vi "test_Create MetaData Channel_array enumerated list.vi"(8 "error in (no error)":errorcluster, 11 "TestCase in":refnum<class "Instrument Addon Scripting API Channels Unit Tests.lvclass">) -> (0 "error out":errorcluster, 3 "TestCase out":refnum<class "Instrument Addon Scripting API Channels Unit Tests.lvclass">)   [LabVIEW 2019, in "Instrument Addon Scripting API Channels Unit Tests.lvclass"]
uses:
  Instrument Addon Scripting API Channels Unit Tests.lvclass
  Addon/Addon Shared/Types/FG Control.ctl
  APIs/Scripting API/TypeDefs/Array Enumerated List Settings.ctl
  APIs/Scripting API/TypeDefs/Array Element.ctl
  Instrument Addon Scripting API Channels Unit Tests.lvclass/Instrument Addon Scripting API Channels Unit Tests.ctl
  Addon/Addon Shared/SubVIs/Constants.vi
  <vilib>/NI VeriStand/Custom Device Tools/Custom Device Utility Library/NI VeriStand - Search for Item by Name.vi
  <vilib>/NI VeriStand/Custom Device API/NI VeriStand - Get Item Property.vi
  <vilib>/NI VeriStand/Custom Device API/Get Item Property (U32).vi
  <vilib>/NI VeriStand/Custom Device API/Get Item Property (String Array).vi
  <vilib>/NI VeriStand/Custom Device API/Get Item Property (String).vi
  <vilib>/NI VeriStand/Custom Device API/NI VeriStand - Set Item Property.vi
  <vilib>/NI VeriStand/Custom Device API/Set Item Property (U32).vi
  <vilib>/NI VeriStand/Custom Device API/Set Item Property (String Array).vi
  <vilib>/NI VeriStand/Custom Device API/NI VeriStand - Get Item Children.vi
  Addon/Addon Shared/SubVIs/Set Channel Value Table.vi
  <vilib>/NI VeriStand/Custom Device API/Set Item Property (String).vi
  <vilib>/NI VeriStand/Custom Device Tools/Custom Device Utility Library/NI VeriStand - Search for Item by GUID.vi
  APIs/Scripting API/Channels/Create MetaData Channel - Array - Enumerated List.vi
  <vilib>/addons/_JKI Toolkits/VI Tester/TestCase.llb/TestCase.lvclass
  <vilib>/NI VeriStand/Custom Device Tools/Custom Device Utility Library/Custom Device Utility Library.lvlib
  Addon/Addon Shared/Instrument Addon Shared.lvlib
  APIs/Scripting API/Instrument Addon Scripting API.lvlib
  C:/Program Files (x86)/National Instruments/LabVIEW 2019/vi.lib/addons/_JKI Toolkits/VI Tester/TestCase.llb/TestCase.lvclass
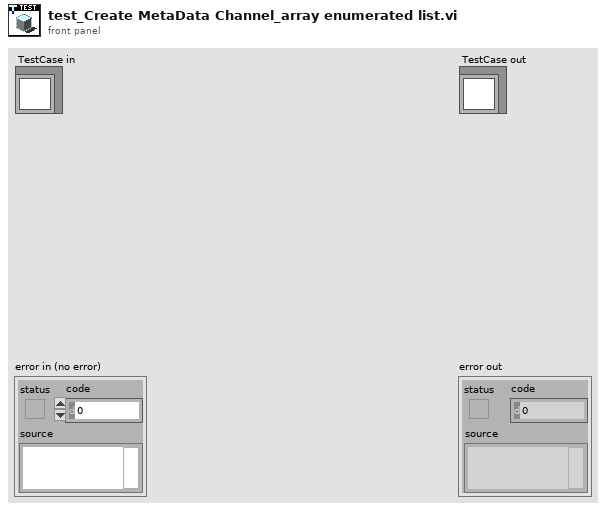
[diagram p1: front panel]
types:
  T1 = typedef "Instrument Addon Shared.lvlib/FG Control.ctl" = enum16{"Get", "Set"}
  T2 = typedef "Instrument Addon Scripting API.lvlib/Array Enumerated List Settings.ctl" = cluster{"Elements":T3[], "Enumerated List":string[], "Delimiter":string}
  T3 = typedef "Instrument Addon Scripting API.lvlib/Array Element.ctl" = cluster{"Name":string, "Default Value":dbl, "Units":string}
  T4 = typedef "Custom Device API.lvlib/Custom Device Item Ref.ctl" = u64
  T5 = typedef "Instrument Addon Shared.lvlib/MetaData Parameters.ctl" = cluster{"Data Type":T6, "Channel Type":T7, "List":string[], "Format String":string, "Type":T8, "Delimiter":string, "Endian":T9}
  T6 = typedef "Instrument Addon Shared.lvlib/Protocol Data Type.ctl" = enum16{"Single Channel", "Array"}
  T7 = typedef "Instrument Addon Shared.lvlib/Metadata Channel Type.ctl" = enum16{"Enumerated List", "Format", "Type Cast"}
  T8 = typedef "Instrument Addon Shared.lvlib/Type Cast Type.ctl" = enum16{"DBL", "SGL", "U64", "U32", "U16", "U8", "I64", "I32", "I16", "I8"}
  T9 = typedef "Instrument Addon Shared.lvlib/Endian.ctl" = enum16{"Native", "Little", "Big"}
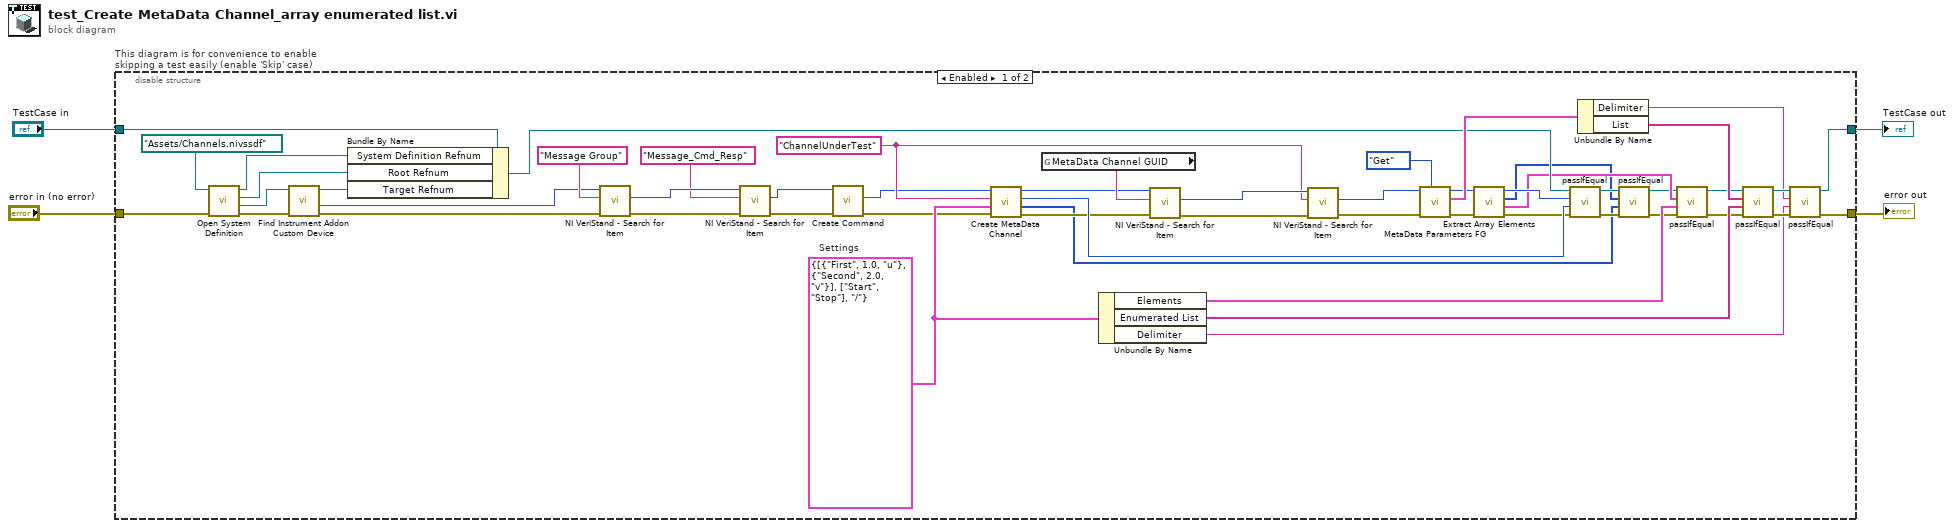
[diagram p0: block diagram]
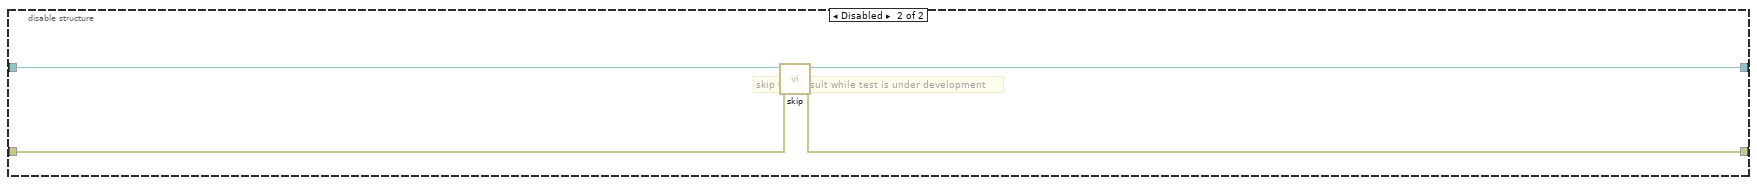
[diagram p2: hidden frame]
diagram:
  n1 = disable-structure "This diagram is for convenience to enable skipping a test easily (enable 'Skip' case)" shown="Enabled" {
    disable-tunnel: "TestCase in" -> [w39 w61]
    disable-tunnel: [w31 w59] -> w1
    disable-tunnel: [w30 w60] -> w3
    disable-tunnel: "error in (no error)" -> [w57 w58]
    frame Enabled {
      w34 = T2 {"Elements"=[{"Name"="First", "Default Value"=1.0, "Units"="u"}, {"Name"="Second", "Default Value"=2.0, "Units"="v"}], "Enumerated List"=["Start", "Stop"], "Delimiter"="/"}  # Settings
      w38 = "ChannelUnderTest" ("Name")
      n2 = call "Open System Definition.vi"("error in (no error)"=w57, "System Definition File"=path "Assets/Channels.nivssdf") -> ("error out"=w55:errorcluster, "Target Refnum"=w56:refnum<k24>, "Root Refnum"=w42:refnum<k24>, "System Definition Refnum"=w41:refnum<k24>)  [unwired: 6 in]
      n3 = call "Find Instrument Addon Custom Device.vi"("error in"=w55, "target in"=w56) -> ("error out"=w17:errorcluster, "NodeID"=w18:u64, "target out"=w43:refnum<k24>)  [unwired: 7 in]
      n4 = Bundle By Name(cluster=w39, "System Definition Refnum"=w41, "Root Refnum"=w42, "Target Refnum"=w43) -> (w40:refnum<class "Instrument Addon Scripting API Channels Unit Tests.lvclass">)
      n5 = call-poly <vilib>:"NI VeriStand - Search for Item.vi"("error in"=w17, "Item Name"="Message Group", "Section Ref in"=w18) -> ("error out"=w19:errorcluster, "Item Ref"=w21:T4)  [unwired: 5 in, 2 out]
      n6 = call-poly <vilib>:"NI VeriStand - Search for Item.vi"("error in"=w19, "Item Name"="Message_Cmd_Resp", "Section Ref in"=w21) -> ("error out"=w8:errorcluster, "Item Ref"=w7:T4)  [unwired: 5 in, 2 out]
      n7 = call "Create Command.vi"("error in"=w8, "message refnum In"=w7) -> ("error out"=w5:errorcluster, "command refnum"=w6:T4)  [unwired: 7 in, 1 out]
      n8 = call-poly "Create MetaData Channel.vi"("error in (no error)"=w5, "settings"=w34, "channel name"=w38, "command refnum in"=w6) -> ("error out"=w35:errorcluster, "channel refnums"=w10:T4[], "array refnum"=w36:T4, "command refnum out"=w37:T4)  [unwired: 4 in]
      n9 = global read "Constants.vi" "MetaData Channel GUID"() -> (w54:string)
      n10 = Unbundle By Name(w34) -> ("Elements"=w27:T3[], "Enumerated List"=w44:string[], "Delimiter"=w33:string)
      n11 = call-poly <vilib>:"NI VeriStand - Search for Item.vi"("error in"=w35, "Item GUID"=w54, "Section Ref in"=w37) -> ("error out"=w52:errorcluster, "Item Ref"=w53:T4)  [unwired: 5 in, 2 out]
      n12 = call-poly <vilib>:"NI VeriStand - Search for Item.vi"("error in"=w52, "Item Name"=w38, "Section Ref in"=w53) -> ("error out"=w51:errorcluster, "Item Ref"=w50:T4)  [unwired: 5 in, 2 out]
      n13 = call "MetaData Parameters FG.vi"("Action"=FG_Control."Get", "error in (no error)"=w51, "Item Ref in"=w50) -> ("error out"=w26:errorcluster, "MetaData Parameters"=w48:T5, "Item Ref out"=w25:T4)  [unwired: 6 in]
      n14 = call "Extract Array Elements.vi"("error in (no error)"=w26, "array reference in"=w25) -> ("error out"=w24:errorcluster, "elements"=w16:T3[], "channel refnums"=w11:T4[], "array reference out"=w23:T4)  [unwired: 6 in]
      n15 = call-dynamic "passIfEqual.vi"("error in (no error)"=w24, "y"=w36, "x"=w23, "TestCase in"=w40) -> ("error out"=w14:errorcluster, "TestCase out"=w15:refnum<class "Instrument Addon Scripting API Channels Unit Tests.lvclass">)  [unwired: 6 in]
      n16 = Unbundle By Name(w48) -> ("Delimiter"=w32:string, "List"=w45:string[])
      n17 = call-dynamic "passIfEqual.vi"("error in (no error)"=w14, "y"=w10, "x"=w11, "TestCase in"=w15) -> ("error out"=w13:errorcluster, "TestCase out"=w12:refnum<class "Instrument Addon Scripting API Channels Unit Tests.lvclass">)  [unwired: 6 in]
      n18 = call-dynamic "passIfEqual.vi"("error in (no error)"=w13, "y"=w27, "x"=w16, "TestCase in"=w12) -> ("error out"=w28:errorcluster, "TestCase out"=w29:refnum<class "Instrument Addon Scripting API Channels Unit Tests.lvclass">)  [unwired: 6 in]
      n19 = call-dynamic "passIfEqual.vi"("error in (no error)"=w28, "y"=w44, "x"=w45, "TestCase in"=w29) -> ("error out"=w47:errorcluster, "TestCase out"=w46:refnum<class "Instrument Addon Scripting API Channels Unit Tests.lvclass">)  [unwired: 6 in]
      n20 = call-dynamic "passIfEqual.vi"("error in (no error)"=w47, "y"=w33, "x"=w32, "TestCase in"=w46) -> ("error out"=w30:errorcluster, "TestCase out"=w31:refnum<class "Instrument Addon Scripting API Channels Unit Tests.lvclass">)  [unwired: 6 in]
    }
    frame Disabled {
      # "skip test result while test is under development"
      n21 = call <vilib>:"skip.vi"("error in (no error)"=w58, "TestCase in"=w61) -> ("error out"=w60:errorcluster, "TestCase out"=w59:refnum<class "Instrument Addon Scripting API Channels Unit Tests.lvclass">)  [unwired: 8 in]
    }
  }
  "error out" <- w3
  "TestCase out" <- w1
